vi "Parse Import String.vi"(8 "error in (no error)":errorcluster, 10 "Raw Segment":T1, 11 "ProtoParser in":refnum<class "ProtoParser.lvclass">) -> (0 "error out":errorcluster, 2 "Import String":string, 3 "ProtoParser out":refnum<class "ProtoParser.lvclass">)   [LabVIEW 2020, in "LV-Protoc.lvlib" / "ProtoParser.lvclass"]
uses:
  ProtoParser.lvclass
  Raw Segment.ctl
  Segment Type.ctl
  Strip To.vi
  LV-Protoc.lvlib
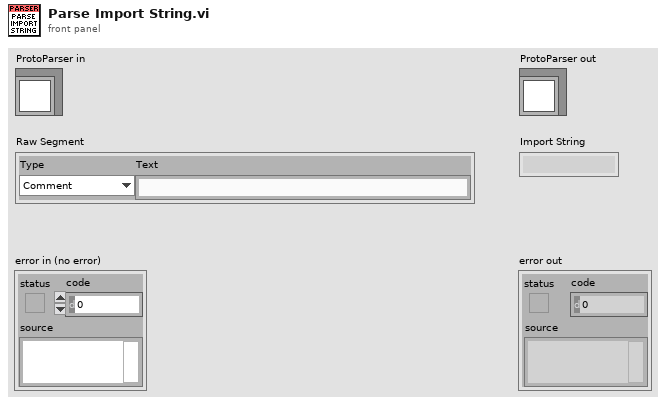
[diagram p1: front panel]
types:
  T1 = typedef "LV-Protoc.lvlib/Raw Segment.ctl" = cluster{"Type":T2, "Text":string}
  T2 = typedef "LV-Protoc.lvlib/Segment Type.ctl" = enum16{"Comment", "Message Open", "Enum Open", "Message Close", "Enum Close", "Field", "Syntax", "Import", "Enum Value", "Package", "Reserved"}
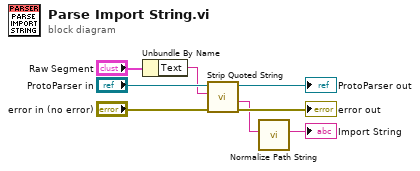
[diagram p0: block diagram]
diagram:
  n1 = Unbundle By Name("Raw Segment") -> ("Text"=w5:string)
  n2 = call "Strip Quoted String.vi"("error in (no error)"="error in (no error)", "Text"=w5, "ProtoParser in"="ProtoParser in") -> ("error out"=→"error out":errorcluster, "String Contents"=w4:string, "ProtoParser out"=→"ProtoParser out":refnum<class "ProtoParser.lvclass">)  [unwired: 5 in, 1 out]
  n3 = call "Normalize Path String.vi"("Import String"=w4) -> ("Normalized Path"=→"Import String":string)  [unwired: 10 in]
